vi "Read I64 Direct.vi"(8 "error in (no error)":errorcluster, 9 "Timeout (ms)":i32, 11 "CIFTag in":refnum<class "CIF_CIPC_Chn_I64.lvclass">) -> (0 "error out":errorcluster, 1 "timed out?":bool, 2 "Data":i64, 3 "CIFTag out":refnum<class "CIF_CIPC_Chn_I64.lvclass">)   [LabVIEW 2021, in "CIF_CIPC_Chn_I64.lvclass"]
uses:
  CIF_CIPC_Chn_I64.lvclass
  D:/dev/Packages/CIF_Channels_Core/src/CIFChannels/CIFChannels.lvclass
  D:/dev/Packages/CIF_Channels_Core/src/CIPC_Channels/CIF_CIPC_Chan/CIF_CIPC_Chn.lvclass
  CIFChannels/CIFChannels.lvclass/CIFChannels.ctl
  CIFChannels/Typedef/Channel State.ctl
  CIFChannels/Typedef/Direction.ctl
  CIF_CIPC_Chn_I64.lvclass/CIF_CIPC_Chn_I64.ctl
  CIF_CIPC_Chan/CIF_CIPC_Chn.lvclass/CIF_CIPC_Chn.ctl
  <vilib>/CIF Foundation/CIF CIPC/TypeDefs/Data Element Details.ctl
  CIF_CIPC_Chan/Accessors/Read Buffer Configuration.vi
  CIF_CIPC_Chan/Accessors/Read Data Type.vi
  CIFChannels/Accessors/Read Channel State.vi
  CIFChannels/Accessors/Read Direction.vi
  CIFChannels/Accessors/Read Tag Forced.vi
  CIFChannels/Accessors/Write Channel State.vi
  CIFChannels/Accessors/Read Tag Disconnect Behavior.vi
  <vilib>/CIF Foundation/CIF CIPC/SubVIs/Wait For N Elements Available.vi
  <vilib>/CIF Foundation/CIF CIPC/SubVIs/Get Element Read Position.vi
  <vilib>/CIF Foundation/CIF CIPC/SubVIs/Check Error.vi
  <vilib>/CIF Foundation/CIF CIPC/SubVIs/Get dll Path.vi
  <vilib>/CIF Foundation/CIF CIPC/SubVIs/Set Element Read Position.vi
  CIF_CIPC_Chan/CIF_CIPC_Chn.lvclass
  <vilib>/Utility/error.llb/Trim Whitespace.vi
  <vilib>/Utility/error.llb/Error Cluster From Error Code.vi
  CIFChannels/CIFChannels.lvclass
  <vilib>/CIF Foundation/CIF CIPC/CIF_NI_CIPC.lvlib
  ba6fad66-2141-4b71-a182-0ba93d8ec932.vi
  415d2b66-d823-4a9e-9883-6ce4ff09bb89.vi
  a3cbe5e6-52fe-4e96-a200-f4d10a132430.vi
  4f1ce4a2-398b-4c7d-a883-0791825cd36c.vi
  abd07148-a4a6-4410-b026-c43785a1b898.vi
  4490a905-f773-409b-91f2-43bf35d7d2a1.vi
  3f7db7d7-f5dc-4da3-aa4d-553df7ca8e68.vi
  8b59d1f9-59b0-43f5-8f44-95e4d5ea48f6.vi
  fcc006bd-2ff1-4888-bcf8-1fe400acd3ba.vi
  0b12b1be-38c7-44d2-80b3-7b2a3ddc6c89.vi
  ea5923f1-9610-4302-a27b-212c9360a415.vi
  8c001dc6-46a3-46ae-82cb-8eb11a864445.vi
  D:/dev/Packages/CIF_Channels_Core/src/CIPC_Channels/I64/CIF_CIPC_Chn_I64.lvclass
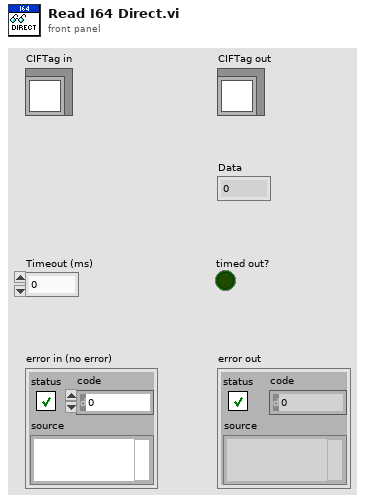
[diagram p1: front panel]
types:
  T1 = typedef "CIFChannels.lvclass/Channel State.ctl" = enum16{"Creating", "Disconnected", "Connecting", "Connected", "Destroyed"}
  T2 = typedef "CIFChannels.lvclass/Direction.ctl" = enum16{"Publisher", "Subscriber"}
  T3 = typedef "CIF_NI_CIPC.lvlib/Data Element Details.ctl" = cluster{"Bytes to Read":u32, "Element Offset":u32}
  T4 = typedef "CIF_CIPC_Chn.lvclass/Buffer Configuration Data.ctl" = cluster{"Total Size":u32, "Read Size":u32, "Read Offset":u32, "CIPC BP References":T5, "Override CIPC Name":string, "Encoder Data":string}
  T5 = typedef "CIF_NI_CIPC.lvlib/Backpressure References.ctl" = cluster{"CIPC Reference":u64, "CIPC BP Reference":u64}
  T6 = typedef "NI_Data Type.lvlib/Data Type.ctl" = enum8{"Invalid Type", "Void", "I8", "I16", "I32", "I64", "U8", "U16", "U32", "U64", "Single Float", "Double Float", "Extended Float", "Single Complex", "Double Complex", "Extended Complex", "Enum U8", "Enum U16", "Enum U32", "Enum U64", "Single Float With Unit", "Double Float With Unit", "Extended Float With Unit", "Single Complex with Unit", "Double Complex with Unit", "Extended Complex with Unit", "Boolean", "String", "Path", "Picture", "Tag", "Array", "Cluster", "Variant", "LV Variant", "Waveform", "Timestamp", "Digital Waveform", "Digital Data", "ExpressData", "Refnum", "External Data", "VI", "Poly VI", "LabVIEW Class Instance", "Fixed Point", "Set Collection", "Map Collection"}
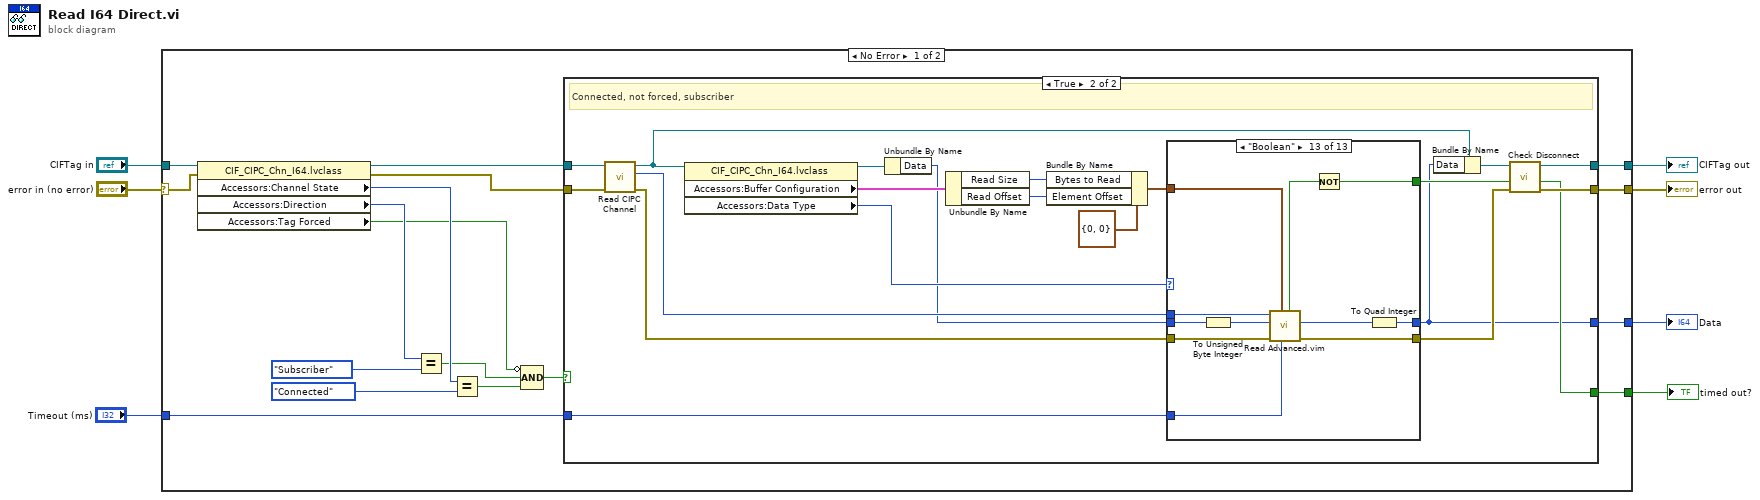
[diagram p0: block diagram]
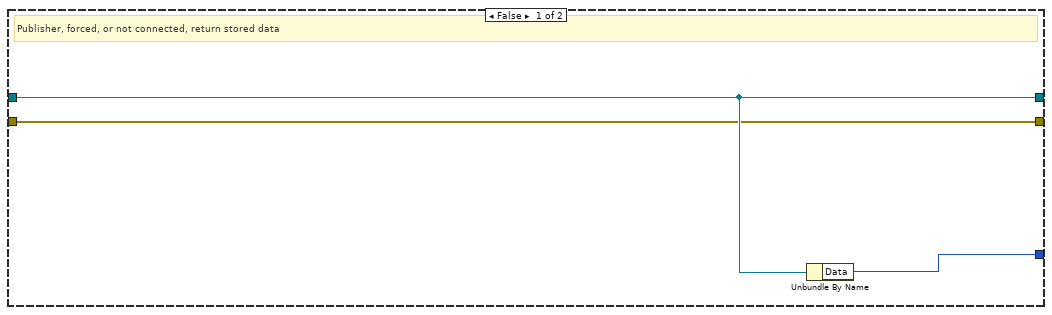
[diagram p2: hidden frame]
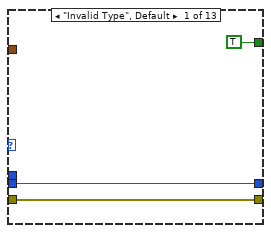
[diagram p3: hidden frame]
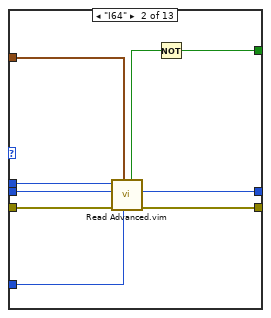
[diagram p4: hidden frame]
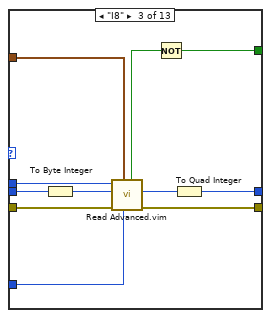
[diagram p5: hidden frame]
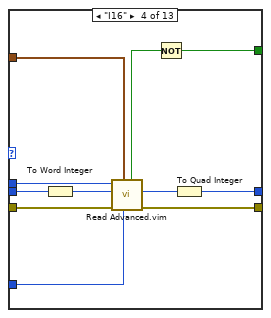
[diagram p6: hidden frame]
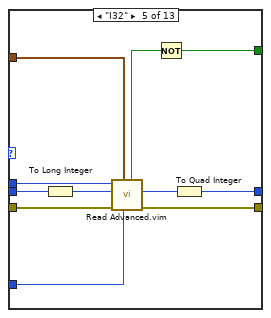
[diagram p7: hidden frame]
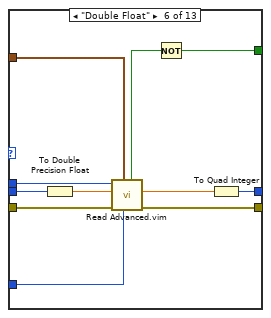
[diagram p8: hidden frame]
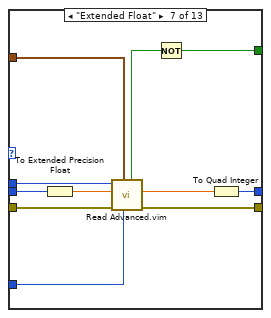
[diagram p9: hidden frame]
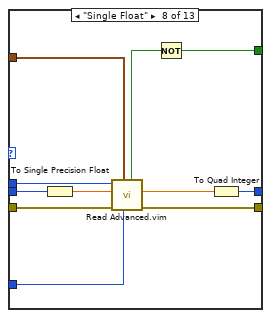
[diagram p10: hidden frame]
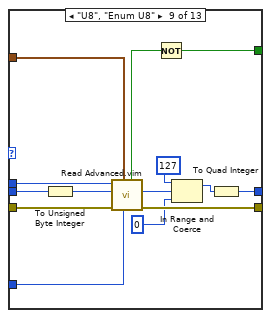
[diagram p11: hidden frame]
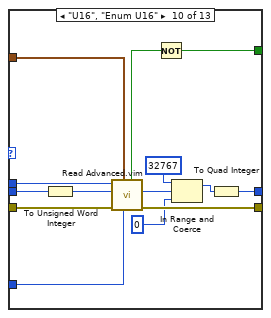
[diagram p12: hidden frame]
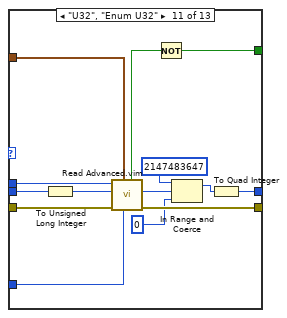
[diagram p13: hidden frame]
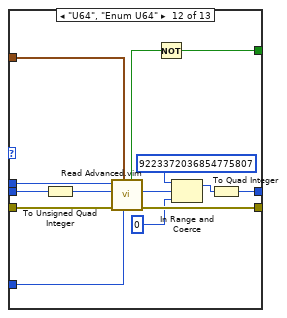
[diagram p14: hidden frame]
diagram:
  n1 = case shown="No Error" "error in (no error)" {
    selector: "error in (no error)" -> [w21 w195]
    tunnel: [w10 w195] -> w6
    tunnel: [w11 w194] -> w4
    tunnel: "CIFTag in" -> [w22 w194]
    tunnel: [w24 _] -> w3
    tunnel: [w23 _] -> w2
    tunnel: "Timeout (ms)" -> [w9 _]
    frame No Error {
      n2 = property class="CIF_CIPC_Chn_I64.lvclass"(reference=w22, error in=w21) -> (reference out=w20:refnum<class "CIF_CIPC_Chn_I64.lvclass">, error out=w19:errorcluster, "Accessors:Channel State"=w16:T1, "Accessors:Direction"=w18:T2, "Accessors:Tag Forced"=w8:bool)
      n3 = Equal?(x=w18, y=Direction."Subscriber") -> (x = y?=w12:bool)
      n4 = Equal?(x=w16, y=Channel_State."Connected") -> (x = y?=w14:bool)
      n5 = Compound Arithmetic op=AND(invert w8, w12, w14) -> (w13:bool)
      n6 = case shown="True" w13 {
        tunnel: [_ w43] -> w24
        tunnel: [w27 w28] -> w23
        tunnel: w19 -> [w25 w47]
        tunnel: w20 -> [w26 w48]
        tunnel: [w26 w45] -> w11
        tunnel: [w25 w46] -> w10
        tunnel: w9 -> [_ w31]
        frame False {
          # "Publisher, forced, or not connected, return stored data"
          n7 = Unbundle By Name(w26) -> ("Data"=w27:i64)
        }
        frame True {
          # "Connected, not forced, subscriber"
          n8 = call "Read CIPC Channel.vi"("error in (no error)"=w47, "CIFTag in"=w48) -> ("error out"=w32:errorcluster, "CIPC Channel"=w34:u64, "CIFTag out"=w42:refnum<class "CIF_CIPC_Chn_I64.lvclass">)  [unwired: 7 in]
          n9 = property class="CIF_CIPC_Chn_I64.lvclass"(reference=w42) -> (reference out=w41:refnum<class "CIF_CIPC_Chn_I64.lvclass">, "Accessors:Buffer Configuration"=w37:T4, "Accessors:Data Type"=w35:T6)  [unwired: 1 in, 1 out]
          n10 = Unbundle By Name(w41) -> ("Data"=w33:i64)
          n11 = Unbundle By Name(w37) -> ("Read Size"=w39:u32, "Read Offset"=w38:u32)
          n12 = Bundle By Name(cluster=T3 {"Bytes to Read"=0, "Element Offset"=0} ("Data Element"), "Bytes to Read"=w39, "Element Offset"=w38) -> (w36:T3)
          n13 = case shown="\"Boolean\"" w35 {
            tunnel: [TRUE w60 w71 w82 w93 w104 w115 w126 w140 w154 w168 w182 w193] -> w29
            tunnel: w36 -> [_ w59 w70 w81 w92 w103 w114 w125 w139 w153 w167 w181 w192]
            tunnel: w34 -> [_ w58 w69 w80 w91 w102 w113 w124 w138 w152 w166 w180 w191]
            tunnel: w32 -> [w50 w57 w68 w79 w90 w101 w112 w123 w137 w151 w165 w179 w190]
            tunnel: w31 -> [_ w56 w67 w78 w89 w100 w111 w122 w136 w150 w164 w178 w189]
            tunnel: [w51 w54 w61 w72 w83 w95 w106 w117 w131 w145 w159 w173 w185] -> w28
            tunnel: w33 -> [w51 w53 w64 w75 w86 w98 w109 w120 w134 w148 w162 w176 w187]
            tunnel: [w50 w52 w63 w74 w85 w97 w108 w119 w133 w147 w161 w175 w186] -> w30
            frame "Invalid Type", Default {
            }
            frame "I64" {
              n14 = call "Read Advanced.vim"("Timeout (ns)"=w56, "Data Element"=w59, "error in (no error)"=w57, "Data in"=w53, "CIPC Reference in"=w58) -> ("error out"=w52:errorcluster, "Data out"=w54:i64, "Success"=w55:bool)  [unwired: 2 in, 2 out]
              n15 = Not(x=w55) -> (.not. x?=w60:bool)
            }
            frame "I8" {
              n16 = To Byte Integer(number=w64) -> (8bit integer=w62:i8)
              n17 = call "Read Advanced.vim"("Timeout (ns)"=w67, "Data Element"=w70, "error in (no error)"=w68, "Data in"=w62, "CIPC Reference in"=w69) -> ("error out"=w63:errorcluster, "Data out"=w65:i8, "Success"=w66:bool)  [unwired: 2 in, 2 out]
              n18 = Not(x=w66) -> (.not. x?=w71:bool)
              n19 = To Quad Integer(1:w65) -> (0:w61:i64)
            }
            frame "I16" {
              n20 = To Word Integer(number=w75) -> (16bit integer=w73:i16)
              n21 = call "Read Advanced.vim"("Timeout (ns)"=w78, "Data Element"=w81, "error in (no error)"=w79, "Data in"=w73, "CIPC Reference in"=w80) -> ("error out"=w74:errorcluster, "Data out"=w76:i16, "Success"=w77:bool)  [unwired: 2 in, 2 out]
              n22 = Not(x=w77) -> (.not. x?=w82:bool)
              n23 = To Quad Integer(1:w76) -> (0:w72:i64)
            }
            frame "I32" {
              n24 = To Long Integer(number=w86) -> (32bit integer=w84:i32)
              n25 = call "Read Advanced.vim"("Timeout (ns)"=w89, "Data Element"=w92, "error in (no error)"=w90, "Data in"=w84, "CIPC Reference in"=w91) -> ("error out"=w85:errorcluster, "Data out"=w87:i32, "Success"=w88:bool)  [unwired: 2 in, 2 out]
              n26 = Not(x=w88) -> (.not. x?=w93:bool)
              n27 = To Quad Integer(1:w87) -> (0:w83:i64)
            }
            frame "Double Float" {
              n28 = To Double Precision Float(number=w98) -> (double precision float=w96:dbl)
              n29 = call "Read Advanced.vim"("Timeout (ns)"=w100, "Data Element"=w103, "error in (no error)"=w101, "Data in"=w96, "CIPC Reference in"=w102) -> ("error out"=w97:errorcluster, "Data out"=w94:dbl, "Success"=w99:bool)  [unwired: 2 in, 2 out]
              n30 = Not(x=w99) -> (.not. x?=w104:bool)
              n31 = To Quad Integer(1:w94) -> (0:w95:i64)
            }
            frame "Extended Float" {
              n32 = To Extended Precision Float(1:w109) -> (0:w107:ext)
              n33 = call "Read Advanced.vim"("Timeout (ns)"=w111, "Data Element"=w114, "error in (no error)"=w112, "Data in"=w107, "CIPC Reference in"=w113) -> ("error out"=w108:errorcluster, "Data out"=w105:ext, "Success"=w110:bool)  [unwired: 2 in, 2 out]
              n34 = Not(x=w110) -> (.not. x?=w115:bool)
              n35 = To Quad Integer(1:w105) -> (0:w106:i64)
            }
            frame "Single Float" {
              n36 = To Single Precision Float(number=w120) -> (single precision float=w118:sgl)
              n37 = call "Read Advanced.vim"("Timeout (ns)"=w122, "Data Element"=w125, "error in (no error)"=w123, "Data in"=w118, "CIPC Reference in"=w124) -> ("error out"=w119:errorcluster, "Data out"=w116:sgl, "Success"=w121:bool)  [unwired: 2 in, 2 out]
              n38 = Not(x=w121) -> (.not. x?=w126:bool)
              n39 = To Quad Integer(1:w116) -> (0:w117:i64)
            }
            frame "U8", "Enum U8" {
              n40 = To Unsigned Byte Integer(number=w134) -> (unsigned 8bit integer=w132:u8)
              n41 = call "Read Advanced.vim"("Timeout (ns)"=w136, "Data Element"=w139, "error in (no error)"=w137, "Data in"=w132, "CIPC Reference in"=w138) -> ("error out"=w133:errorcluster, "Data out"=w130:u8, "Success"=w135:bool)  [unwired: 2 in, 2 out]
              n42 = Not(x=w135) -> (.not. x?=w140:bool)
              n43 = In Range and Coerce(upper limit=u8 127, x=w130, lower limit=u8 0) -> (coerced(x)=w129:u8)  [unwired: 1 out]
              n44 = To Quad Integer(1:w129) -> (0:w131:i64)
            }
            frame "U16", "Enum U16" {
              n45 = To Unsigned Word Integer(number=w148) -> (unsigned 16bit integer=w146:u16)
              n46 = call "Read Advanced.vim"("Timeout (ns)"=w150, "Data Element"=w153, "error in (no error)"=w151, "Data in"=w146, "CIPC Reference in"=w152) -> ("error out"=w147:errorcluster, "Data out"=w144:u16, "Success"=w149:bool)  [unwired: 2 in, 2 out]
              n47 = Not(x=w149) -> (.not. x?=w154:bool)
              n48 = In Range and Coerce(upper limit=u16 32767, x=w144, lower limit=u16 0) -> (coerced(x)=w143:u16)  [unwired: 1 out]
              n49 = To Quad Integer(1:w143) -> (0:w145:i64)
            }
            frame "U32", "Enum U32" {
              n50 = To Unsigned Long Integer(number=w162) -> (unsigned 32bit integer=w160:u32)
              n51 = call "Read Advanced.vim"("Timeout (ns)"=w164, "Data Element"=w167, "error in (no error)"=w165, "Data in"=w160, "CIPC Reference in"=w166) -> ("error out"=w161:errorcluster, "Data out"=w158:u32, "Success"=w163:bool)  [unwired: 2 in, 2 out]
              n52 = Not(x=w163) -> (.not. x?=w168:bool)
              n53 = In Range and Coerce(upper limit=u32 2147483647, x=w158, lower limit=u32 0) -> (coerced(x)=w157:u32)  [unwired: 1 out]
              n54 = To Quad Integer(1:w157) -> (0:w159:i64)
            }
            frame "U64", "Enum U64" {
              n55 = To Unsigned Quad Integer(1:w176) -> (0:w174:u64)
              n56 = call "Read Advanced.vim"("Timeout (ns)"=w178, "Data Element"=w181, "error in (no error)"=w179, "Data in"=w174, "CIPC Reference in"=w180) -> ("error out"=w175:errorcluster, "Data out"=w172:u64, "Success"=w177:bool)  [unwired: 2 in, 2 out]
              n57 = Not(x=w177) -> (.not. x?=w182:bool)
              n58 = In Range and Coerce(upper limit=u64 9223372036854775807, x=w172, lower limit=u64 0) -> (coerced(x)=w171:u64)  [unwired: 1 out]
              n59 = To Quad Integer(1:w171) -> (0:w173:i64)
            }
            frame "Boolean" {
              n60 = To Unsigned Byte Integer(number=w187) -> (unsigned 8bit integer=w184:u8)
              n61 = call "Read Advanced.vim"("Timeout (ns)"=w189, "Data Element"=w192, "error in (no error)"=w190, "Data in"=w184, "CIPC Reference in"=w191) -> ("error out"=w186:errorcluster, "Data out"=w183:u8, "Success"=w188:bool)  [unwired: 2 in, 2 out]
              n62 = Not(x=w188) -> (.not. x?=w193:bool)
              n63 = To Quad Integer(1:w183) -> (0:w185:i64)
            }
          }
          n64 = Bundle By Name(cluster=w42, "Data"=w28) -> (w44:refnum<class "CIF_CIPC_Chn_I64.lvclass">)
          n65 = call "Check Disconnect.vi"("error in (no error)"=w30, "timeout in"=w29, "CIFTag in"=w44) -> ("error out"=w46:errorcluster, "timeout out"=w43:bool, "CIFTag out"=w45:refnum<class "CIF_CIPC_Chn_I64.lvclass">)  [unwired: 5 in, 1 out]
        }
      }
    }
    frame Error {
    }
  }
  "error out" <- w6
  "CIFTag out" <- w4
  "timed out?" <- w3
  "Data" <- w2
